vi "Get Steering Wheel Information.vi"(8 "error in (no error)":errorcluster, 11 "wheel in":refnum<class "NI_Robotics_Wheel.lvclass">) -> (0 "error out":errorcluster, 1 "wheel name":string, 2 "wheel parameters":T3={"wheel radius"=1.0, "gear ratio"=1.0, "forward rotation direction"=0} {"forward rotation direction" items=["Clockwise", "Counterclockwise"]}, 3 "wheel out":refnum<class "NI_Robotics_Wheel.lvclass">, 4 "motor communication":refnum<class "NI_Robotics_Motor Communication.lvclass">, 5 "steering parameters":T1={"steering gear ratio"=1.0, "motor angle offset (rad)"=0.0, "steering angle range"={"min steering angle (rad)"=-3.14159, "max steering angle (rad)"=3.141592653589793}}, 6 "steering motor communication":refnum<class "NI_Robotics_Motor Communication.lvclass">)   [LabVIEW 2017, in "NI_Robotics_Wheel.lvclass"]
doc: "Returns information, such as <B>wheel radius</B> and <B>gear ratio</B>, for the wheel you specify. You must manually select the polymorphic instance to use."
uses:
  <vilib>/robotics/Steering/Wheel/NI_Robotics_Wheel.lvclass
  <vilib>/robotics/Steering/Wheel/Wheel Parameters.ctl
  <vilib>/robotics/Steering/Wheel/Rotation Direction.ctl
  <vilib>/robotics/Actuation/Motor Communication/NI_Robotics_Motor Communication.lvclass
  <vilib>/robotics/Steering/Steering Wheel/Steering Wheel Parameters.ctl
  <vilib>/robotics/Steering/Steering Wheel/Steering Angle Range.ctl
  <vilib>/robotics/Steering/Steering Wheel/NI_Robotics_Steering Wheel.lvclass
  c:/Program Files (x86)/National Instruments/LabVIEW 2017/vi.lib/robotics/Steering/Wheel/NI_Robotics_Wheel.lvclass
  <vilib>/robotics/Steering/Wheel/NI_Robotics_Wheel.lvclass/NI_Robotics_Wheel.ctl
  <vilib>/robotics/Steering/Steering Wheel/NI_Robotics_Steering Wheel.lvclass/NI_Robotics_Steering Wheel.ctl
  <vilib>/robotics/Steering/Wheel/Get Motor Communication.vi
  <vilib>/robotics/Steering/Wheel/Get Wheel Parameters.vi
  <vilib>/robotics/Steering/Steering Wheel/Get Steering Wheel Parameters.vi
  <vilib>/robotics/Utilities/Generate Error.vi
  <vilib>/robotics/Utilities/Clear Specific Error.vi
  <vilib>/Analysis/coordinate.llb/Wrap Angle.vi
  <vilib>/Analysis/coordinate.llb/Wrap Angle (scalar).vi
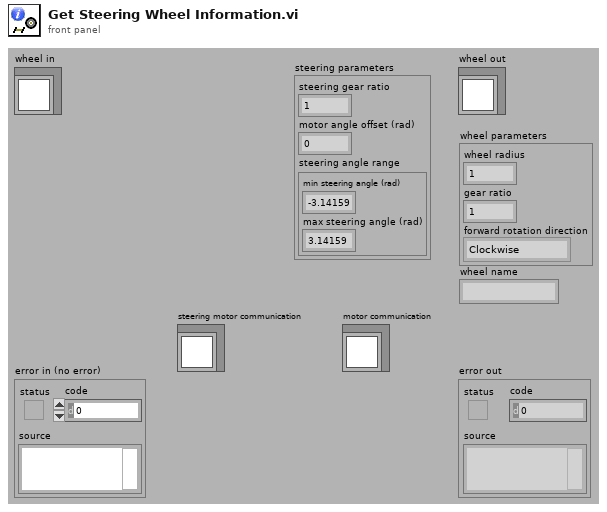
[diagram p1: front panel]
types:
  T1 = typedef "NI_Robotics_Steering Wheel.lvclass/Steering Wheel Parameters.ctl" = cluster{"steering gear ratio":dbl, "motor angle offset (rad)":dbl, "steering angle range":T2}
  T2 = typedef "NI_Robotics_Steering Wheel.lvclass/Steering Angle Range.ctl" = cluster{"min steering angle (rad)":dbl, "max steering angle (rad)":dbl}
  T3 = typedef "NI_Robotics_Wheel.lvclass/Wheel Parameters.ctl" = cluster{"wheel radius":dbl, "gear ratio":dbl, "forward rotation direction":T4}
  T4 = typedef "NI_Robotics_Wheel.lvclass/Rotation Direction.ctl" = u16
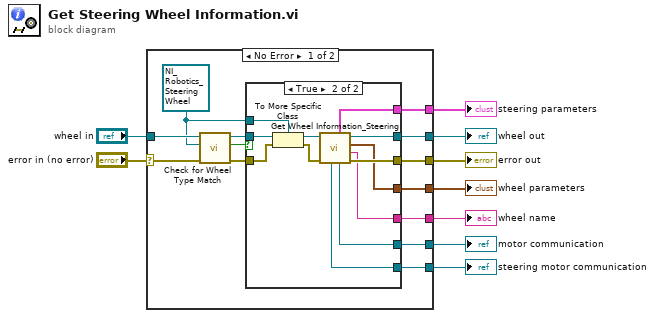
[diagram p0: block diagram]
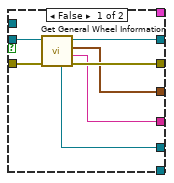
[diagram p2: hidden frame]
diagram:
  n1 = case shown="No Error" "error in (no error)" {
    selector: "error in (no error)" -> [w11 w43]
    tunnel: [w21 w43] -> w8
    tunnel: [w22 w42] -> w6
    tunnel: "wheel in" -> [w15 w42]
    tunnel: [w20 _] -> w5
    tunnel: [w19 _] -> w4
    tunnel: [w18 _] -> w3
    tunnel: [w17 _] -> w2
    tunnel: [w16 _] -> w1
    frame No Error {
      w10 = refnum<class "NI_Robotics_Steering Wheel.lvclass"> refnum ("steering wheel in")
      n2 = call <vilib>:"Check for Wheel Type Match.vi"("error in (no error)"=w11, "target wheel type"=w10, "wheel in"=w15) -> ("error out"=w12:errorcluster, "match?"=w13:bool, "wheel out"=w14:refnum<class "NI_Robotics_Wheel.lvclass">)  [unwired: 6 in]
      n3 = case shown="True" w13 {
        tunnel: w14 -> [w29 w34]
        tunnel: [w26 w41] -> w22
        tunnel: w10 -> [_ w33]
        tunnel: [w27 w40] -> w21
        tunnel: [w25 w39] -> w20
        tunnel: [w24 w38] -> w19
        tunnel: [w23 w37] -> w18
        tunnel: [_ w36] -> w17
        tunnel: [_ w35] -> w16
        tunnel: w12 -> [w28 w31]
        frame False {
          n4 = call <vilib>:"Get General Wheel Information.vi"("error in (no error)"=w28, "wheel in"=w29) -> ("error out"=w27:errorcluster, "wheel name"=w24:string, "wheel parameters"=w25:T3, "wheel out"=w26:refnum<class "NI_Robotics_Wheel.lvclass">, "motor communication"=w23:refnum<class "NI_Robotics_Motor Communication.lvclass">)  [unwired: 5 in]
        }
        frame True {
          n5 = To More Specific Class(target class=w33, reference=w34, error in=w31) -> (specific class reference=w32:refnum<class "NI_Robotics_Steering Wheel.lvclass">, error out=w30:errorcluster)
          n6 = call <vilib>:"Get Wheel Information_Steering.vi"("error in (no error)"=w30, "steering wheel in"=w32) -> ("error out"=w40:errorcluster, "wheel name"=w38:string, "wheel parameters"=w39:T3, "steering wheel out"=w41:refnum<class "NI_Robotics_Steering Wheel.lvclass">, "motor communication"=w37:refnum<class "NI_Robotics_Motor Communication.lvclass">, "steering parameters"=w35:T1, "steering motor communication"=w36:refnum<class "NI_Robotics_Motor Communication.lvclass">)  [unwired: 3 in]
        }
      }
    }
    frame Error {
    }
  }
  "error out" <- w8
  "wheel out" <- w6
  "wheel parameters" <- w5
  "wheel name" <- w4
  "motor communication" <- w3
  "steering motor communication" <- w2
  "steering parameters" <- w1
